vi "Set Channel Redline.vi"(8 "error in (no error)":errorcluster, 9 "Name":string, 10 "Redline":bool, 11 "Channels in":map{string, T1}(c390)) -> (0 "error out":errorcluster, 3 "Channels":map{string, T1}(c390))   [LabVIEW 2020, in "VolatusGUIElements.lvlib" / "BluelinesRedlines.lvclass"]
uses:
  BluelinesRedlines.lvclass
  BluelinesRedlines.lvclass/BluelinesRedlines.ctl
  lv-vecto/Vecto/Channel DBL/Channel DBL.lvclass
  Channel Info.ctl
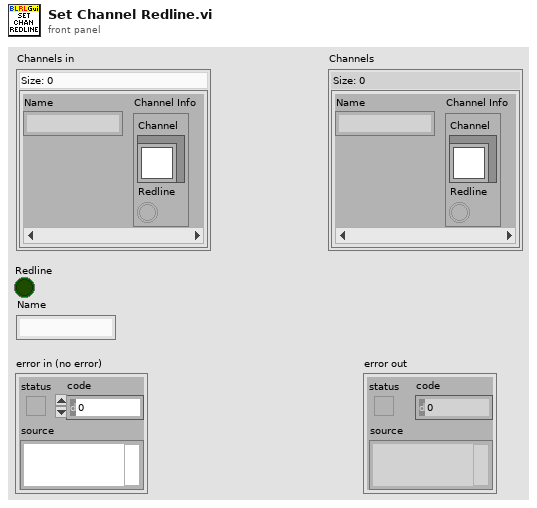
[diagram p1: front panel]
types:
  T1 = typedef "VolatusGUIElements.lvlib/BluelinesRedlines.lvclass/Channel Info.ctl" = cluster{"Channel":refnum<class "Channel DBL.lvclass">, "Redline":bool}
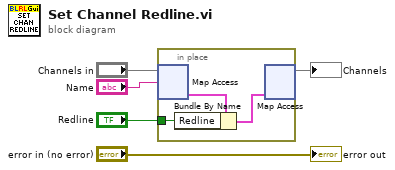
[diagram p0: block diagram]
diagram:
  n1 = in-place {
    in-place-border: "Redline" -> [w7]
    n2 = in-place-map #1("Channels in", "Name") -> (w8:T1)  [unwired: 1 in, 1 out]
    n3 = Bundle By Name(cluster=w8, "Redline"=w7) -> (w6:T1)
    n4 = in-place-map #1(w6) -> (→"Channels":map{string, T1})  [unwired: 1 in, 2 out]
  }
  "error out" <- "error in (no error)"
